vi "Move Up Waveform in List.vi"(7 "Waveform List Ctl Ref":refnum<vi>, 8 "error in (no error)":errorcluster, 11 "Canvas Wfm Array In":waveform(dbl)[](array[waveform])) -> (0 "error out":errorcluster, 3 "Canvas Wfm Array Out":waveform(dbl)[](array[waveform]))   [LabVIEW 2025, in "TDMS Waveform Creator UI.lvlib"]
uses:
  TDMS Waveform Creator UI.lvlib
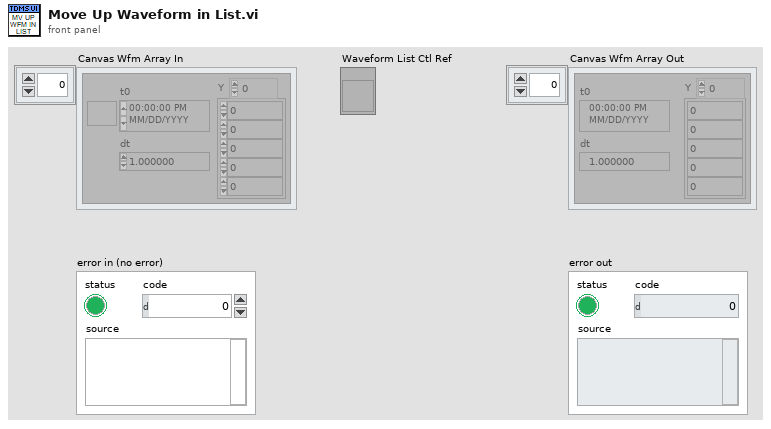
[diagram p1: front panel]
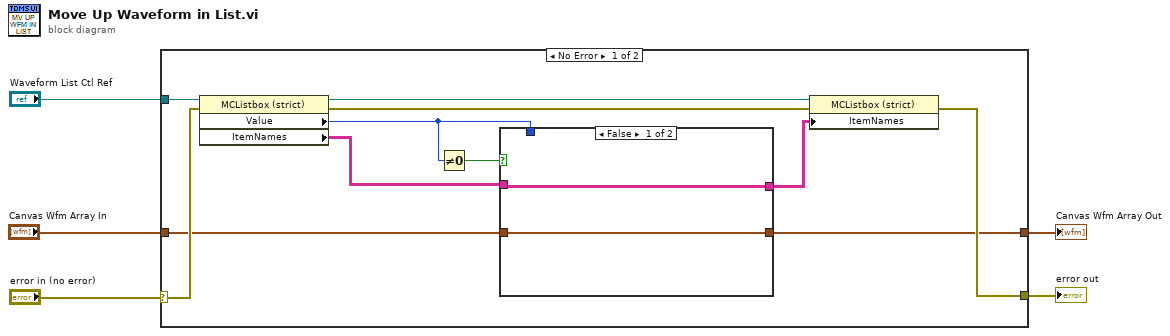
[diagram p0: block diagram]
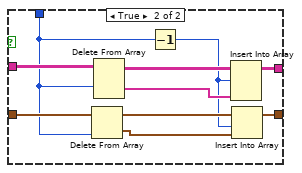
[diagram p2: hidden frame]
diagram:
  n1 = case shown="No Error" "error in (no error)" {
    selector: "error in (no error)" -> [w14 w30]
    tunnel: "Waveform List Ctl Ref" -> [w16 _]
    tunnel: "Canvas Wfm Array In" -> [w10 w29]
    tunnel: [w8 w29] -> w2
    tunnel: [w13 w30] -> w1
    frame No Error {
      n2 = property class="MCListbox (strict)"(reference=w16, error in=w14) -> (reference out=w15:refnum<vi>, error out=w12:errorcluster, "Value"=w7:i32, "ItemNames"=w11:string[][])
      n3 = Not Equal To 0?(x=w7) -> (x != 0?=w6:bool)
      n4 = case shown="False" w6 {
        tunnel: w11 -> [w18 w28]
        tunnel: w10 -> [w17 w25]
        tunnel: w7 -> [_ w24]
        tunnel: [w18 w23] -> w9
        tunnel: [w17 w21] -> w8
        frame False {
        }
        frame True {
          n5 = Delete From Array(array=w25, index=w24) -> (deleted portion=w20:waveform(dbl), array with subset deleted=w27:waveform(dbl)[])  [unwired: 1 in]
          n6 = Delete From Array(array=w28, index (row)=w24) -> (deleted portion=w22:string[], array with subset deleted=w26:string[][])  [unwired: 2 in]
          n7 = Decrement(x=w24) -> (x-1=w19:i32)
          n8 = Insert Into Array(array=w26, index (row)=w19, new element=w22) -> (w23:string[][])  [unwired: 1 in]
          n9 = Insert Into Array(array=w27, index=w19, new element=w20) -> (w21:waveform(dbl)[])
        }
      }
      n10 = property class="MCListbox (strict)"(reference=w15, error in=w12, "ItemNames"=w9) -> (error out=w13:errorcluster)  [unwired: 1 out]
    }
    frame Error {
    }
  }
  "error out" <- w1
  "Canvas Wfm Array Out" <- w2
